vi "Configure Limit Line Testing.vi"(0 "VISA resource name":refnum<visa-resource-name>, 1 "Enable Limit Line Function (F: Disable)":bool, 5 "Line Number (1: Line 1)":i32(ring)=1 items=["Line 1"=1, "Line 2"=2], 7 "Limit Line X-axis Value (0: Frequency)":i32(ring) items=["Frequency", "Time"], 9 "Limit Line Mode (0: Fixed)":i32(ring) items=["Fixed", "Relative"], 11 "error in (no error)":errorcluster, 12 "Enable Limit State (T: Enable)":bool=TRUE) -> (4 "VISA resource name out":refnum<visa-resource-name>, 15 "error out":errorcluster)   [LabVIEW 2022 SP3, in "Agilent N934X Series.lvlib"]
doc: "Configures Limit Line Testing."
uses:
  <instrlib>/Agilent N934X Series/Agilent N934X Series.lvlib
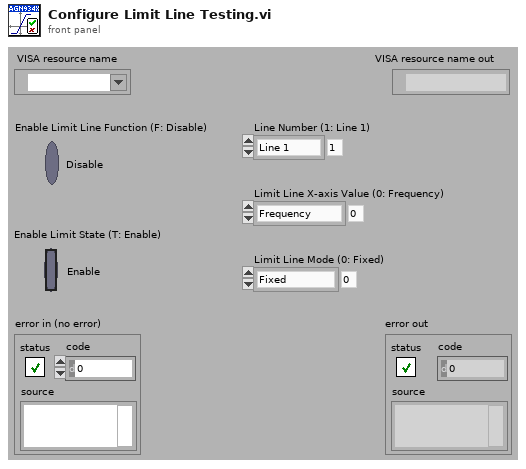
[diagram p1: front panel]
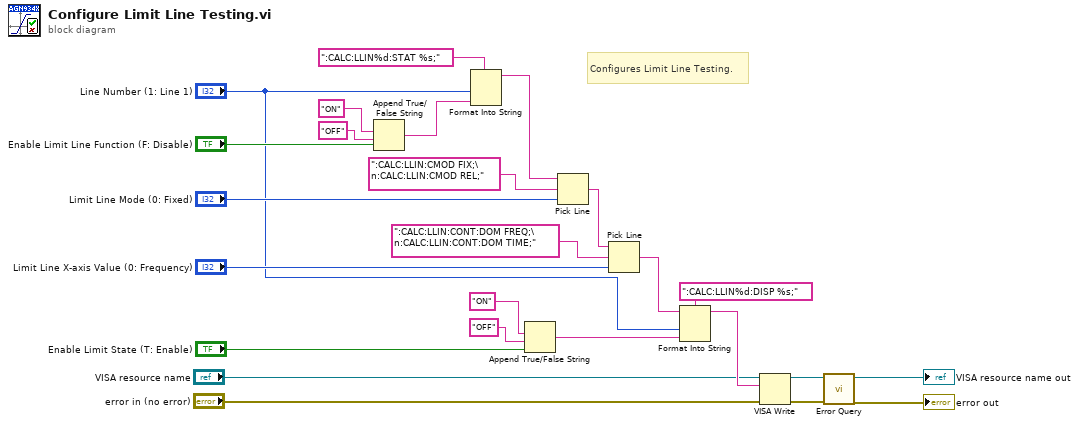
[diagram p0: block diagram]
diagram:
  # "Configures Limit Line Testing."
  n1 = Append True/False String(1:"Enable Limit Line Function (F: Disable)", 2:"OFF", 3:"ON") -> (0:w21:string)  [unwired: 1 in]
  n2 = Format Into String(format string=":CALC:LLIN%d:STAT %s;", "Line Number (1: Line 1)", w21) -> (resulting string=w18:string)  [unwired: 2 in, 1 out]
  n3 = Append True/False String(1:"Enable Limit State (T: Enable)", 2:"OFF", 3:"ON") -> (0:w9:string)  [unwired: 1 in]
  n4 = Pick Line(string ("")=w18, multi-line string=":CALC:LLIN:CMOD FIX;\n:CALC:LLIN:CMOD REL;", line index="Limit Line Mode (0: Fixed)") -> (output string=w15:string)
  n5 = Pick Line(string ("")=w15, multi-line string=":CALC:LLIN:CONT:DOM FREQ;\n:CALC:LLIN:CONT:DOM TIME;", line index="Limit Line X-axis Value (0: Frequency)") -> (output string=w11:string)
  n6 = Format Into String(format string=":CALC:LLIN%d:DISP %s;", initial string=w11, "Line Number (1: Line 1)", w9) -> (resulting string=w8:string)  [unwired: 1 in, 1 out]
  n7 = VISA Write(VISA resource name="VISA resource name", write buffer=w8, error in (no error)="error in (no error)") -> (VISA resource name out=w5:refnum<visa-resource-name>, error out=w4:errorcluster)  [unwired: 1 out]
  n8 = call <instrlib>:"Error Query.vi"("error in (no error)"=w4, "VISA resource name"=w5) -> ("error out"=→"error out":errorcluster, "VISA resource name out"=→"VISA resource name out":refnum<visa-resource-name>)  [unwired: 6 in, 2 out]
